vi "Diagram Node Information.vi"(7 "InnerTerminal in":refnum<vi>[](array[refnum]), 8 "error in (no error)":errorcluster, 10 "Array in":refnum<vi>[](array[refnum]), 11 "Front Tunnels":refnum<vi>[](array[refnum])) -> (0 "error out":errorcluster, 1 "Array":cluster{i32, "ClassName":string}[](array[cluster]), 3 "Array out":T1[](array[typedef]))   [LabVIEW 2020, in "CSM-Helper.lvclass"]
uses:
  CSM-Helper.lvclass
  Typedef/Def-Conncted Information.ctl
  <vilib>/Utility/miscctls.llb/LVPositionTypeDef.ctl
  034a7f1a-ae67-47ea-8f8b-10dc9511b7f6.vi
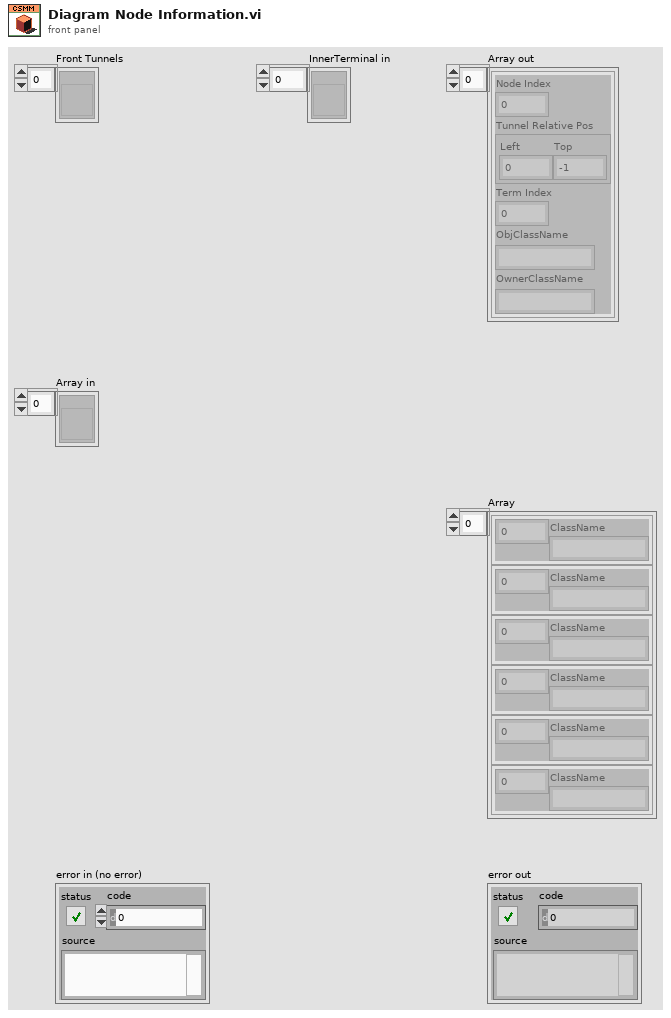
[diagram p1: front panel]
types:
  T1 = typedef "CSM-Helper.lvclass/Def-Conncted Information.ctl" = cluster{"Node Index":i32, "Tunnel Relative Pos":T2, "Term Index":i32, "ObjClassName":string, "OwnerClassName":string}
  T2 = typedef "LVPositionTypeDef.ctl" = cluster{"Left":i32, "Top":i32}
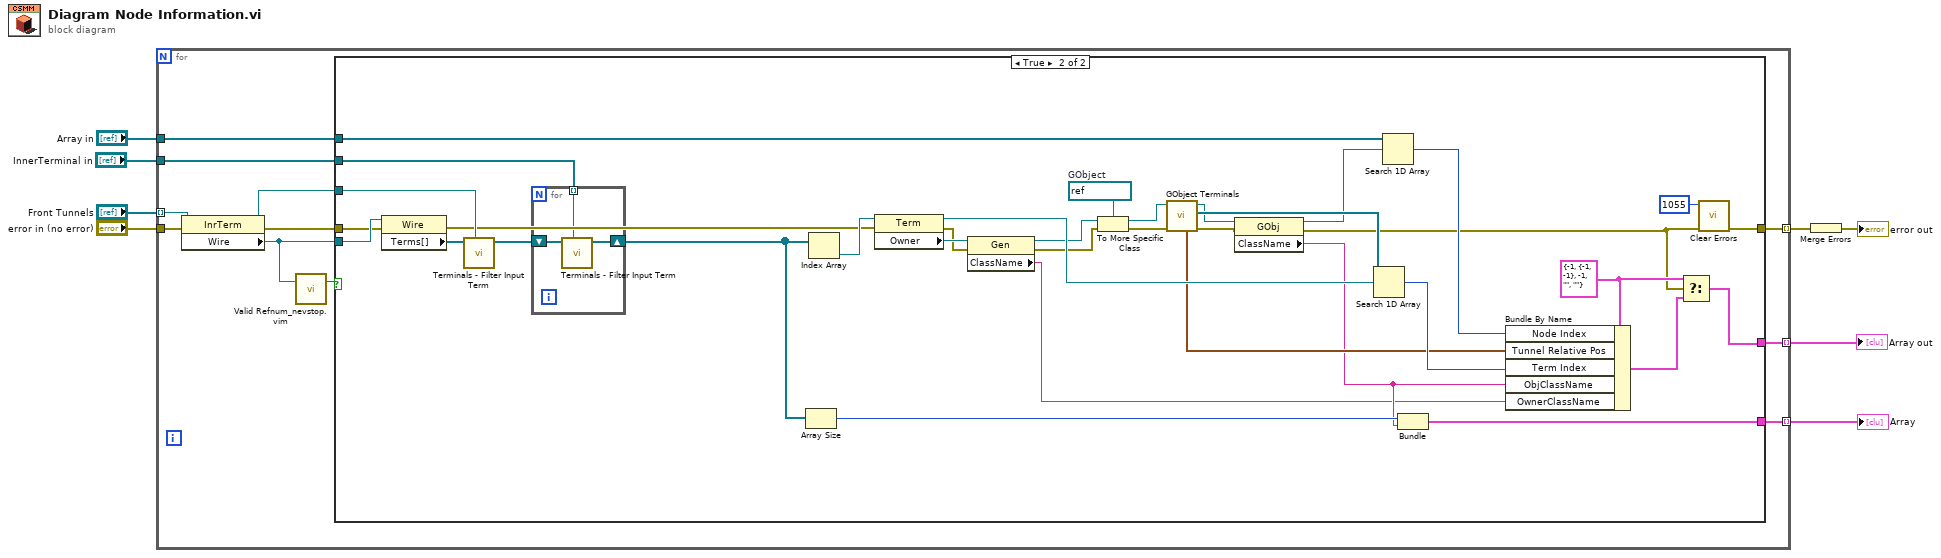
[diagram p0: block diagram]
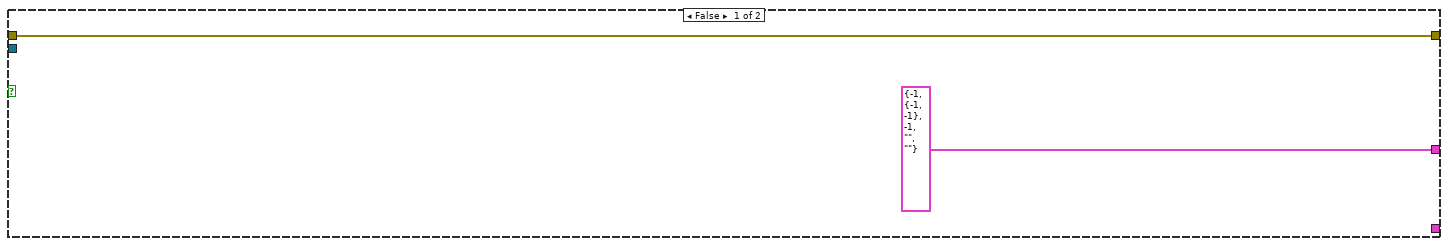
[diagram p2: hidden frame]
diagram:
  n1 = for {
    tunnel: "Array in" -> [w19]
    tunnel: [w13] -> w6 mode=indexing
    tunnel: "Front Tunnels" -> [w18] mode=indexing
    tunnel: "error in (no error)" -> [w17]
    tunnel: [w14] -> w3 mode=indexing
    tunnel: [w10] -> w2 mode=indexing
    tunnel: "InnerTerminal in" -> [w9]
    n2 = property class="InrTerm"(reference=w18, error in=w17) -> (reference out=w15:refnum<vi>, error out=w16:errorcluster, "Wire"=w11:refnum<vi>)
    n3 = call "Valid Refnum_nevstop.vim"("number/path/refnum"=w11) -> ("Valid Number/Path/Refnum"=w12:bool)  [unwired: 2 in]
    n4 = case shown="True" w12 {
      tunnel: w19 -> [_ w46]
      tunnel: w11 -> [_ w56]
      tunnel: w16 -> [w21 w55]
      tunnel: w15 -> [_ w53]
      tunnel: [w21 w49] -> w14
      tunnel: [T1 {"Node Index"=-1, "Tunnel Relative Pos"={"Left"=-1, "Top"=-1}, "Term Index"=-1, "ObjClassName"="", "OwnerClassName"=""} ("cluster") w47] -> w13
      tunnel: [_ w42] -> w10
      tunnel: w9 -> [_ w24]
      frame False {
      }
      frame True {
        w38 = T1 {"Node Index"=-1, "Tunnel Relative Pos"={"Left"=-1, "Top"=-1}, "Term Index"=-1, "ObjClassName"="", "OwnerClassName"=""} ("cluster")
        w45 = refnum<vi> refnum  # GObject
        n5 = property class="Wire"(reference=w56, error in=w55) -> (error out=w51:errorcluster, "Terms[]"=w54:refnum<vi>[])  [unwired: 1 out]
        n6 = call "Terminals - Filter Input Term.vi"("InnerTerminal in"=w53, "Wire.Terms[] in"=w54) -> ("Wire.Terms[] out"=w26:refnum<vi>[])  [unwired: 9 in]
        n7 = for {
          shift-right: [w58] -> w25
          shift-left: w26 -> [w59]
          tunnel: w24 -> [w57] mode=indexing
          n8 = call "Terminals - Filter Input Term.vi"("InnerTerminal in"=w57, "Wire.Terms[] in"=w59) -> ("Wire.Terms[] out"=w58:refnum<vi>[])  [unwired: 9 in]
        }
        n9 = Array Size(array=w25) -> (size(s)=w43:i32)
        n10 = Index Array(array=w25) -> (element=w52:refnum<vi>)  [unwired: 1 in]
        n11 = property class="Term"(reference=w52, error in=w51) -> (reference out=w50:refnum<vi>, error out=w29:errorcluster, "Owner"=w31:refnum<vi>)
        n12 = property class="Gen"(reference=w31, error in=w29) -> (reference out=w30:refnum<vi>, error out=w28:errorcluster, "ClassName"=w27:string)
        n13 = To More Specific Class(target class=w45, reference=w30, error in=w28) -> (specific class reference=w40:refnum<vi>, error out=w41:errorcluster)
        n14 = call "GObject Terminals.vi"("error in (no error)"=w41, "GObject in"=w40) -> ("error in (no error) (dup)"=w23:errorcluster, "Terms[]"=w39:refnum<vi>[], "Node Object"=w34:refnum<vi>, "tunnel Relative Pos"=w35:T2)  [unwired: 5 in, 1 out]
        n15 = property class="GObj"(reference=w34, error in=w23) -> (reference out=w33:refnum<vi>, error out=w22:errorcluster, "ClassName"=w32:string)
        n16 = Search 1D Array(1D array=w39, element=w50) -> (index of element=w36:i32)  [unwired: 1 in]
        n17 = Search 1D Array(1D array=w46, element=w33) -> (index of element=w44:i32)  [unwired: 1 in]
        n18 = Bundle(w43, "ClassName"=w32) -> (w42:cluster{i32, "ClassName":string})  [unwired: 1 in]
        n19 = Bundle By Name(cluster=w38, "Node Index"=w44, "Tunnel Relative Pos"=w35, "Term Index"=w36, "ObjClassName"=w32, "OwnerClassName"=w27) -> (w37:T1)
        n20 = Select(t=w38, s=w22, f=w37) -> (s? t:f=w47:T1)
        n21 = call <vilib>:"Clear Errors.vi"("error in (no error)"=w22, "specific error code to clear (0: all)"=1055) -> ("error out"=w49:errorcluster)  [unwired: 4 in, 1 out]
      }
    }
  }
  "Array out" <- w6
  "Array" <- w2
  n22 = Merge Errors(w3) -> (→"error out":errorcluster)
